vi "lab session 7.3.vi"() -> ()   [LabVIEW 2020]
panel:
  out "square signal":dynamicdata(graph)
  in  "Number of points":dbl
  in  "Numeric":i32
  out "ramp signal":dynamicdata(graph)
  out "constant signal":i32[](graph)
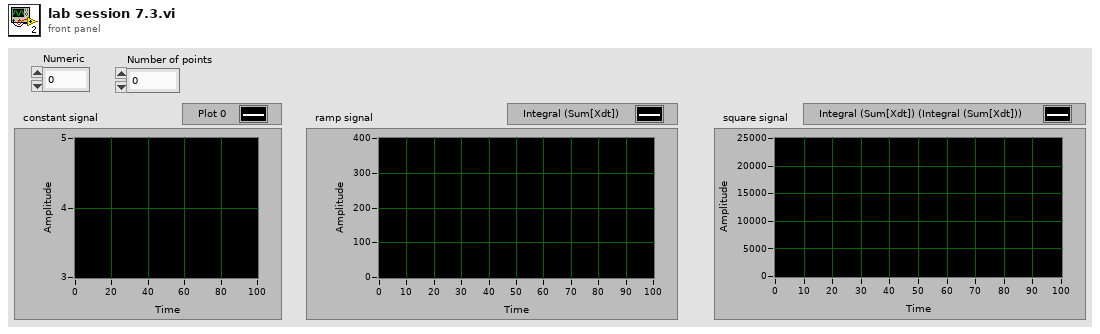
[diagram p1: front panel]
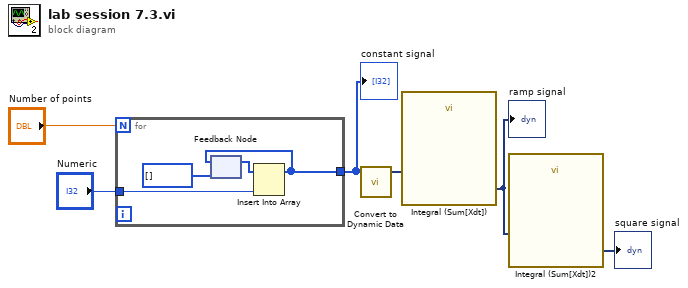
[diagram p0: block diagram]
diagram:
  n1 = for {
    N: "Number of points" -> [_]
    tunnel: [w9] -> w5
    tunnel: "Numeric" -> [w8]
    n2 = feedback #1(i32[] []) -> (w10:i32[])
    n3 = Insert Into Array(array=w10, new element=w8) -> (w9:i32[])  [unwired: 1 in]
    n4 = feedback-in #1(w9) -> ()
  }
  "constant signal" <- w5
  n5 = call "Convert to Dynamic Data"("Array"=w5) -> ("Dynamic Data Type"=w2:dynamicdata)  [unwired: 3 in]
  n6 = call "Integral (Sum[Xdt])"("Signals"=w2) -> ("Result"=w1:dynamicdata)  [unwired: 5 in, 1 out]
  "ramp signal" <- w1
  n7 = call "Integral (Sum[Xdt])2"("Signals"=w1) -> ("Result"=→"square signal":dynamicdata)  [unwired: 5 in, 1 out]
